vi "RenameTerminals.vi"(6 "Dynamic Dispatch":bool, 8 "error in (no error)":errorcluster, 11 "CreateInterface in":refnum<class "CreateInterface.lvclass">) -> (0 "error out":errorcluster)   [LabVIEW 2020, in "Mermaid.lvlib" / "CreateInterface.lvclass"]
uses:
  CreateInterface.lvclass
  CreateInterface.lvclass/CreateInterface.ctl
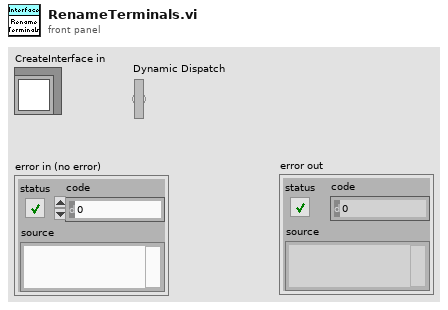
[diagram p1: front panel]
types:
  T1 = enum16{"Invalid Wire Rule", "Required", "Recommended", "Optional", "Dynamic Dispatch"}
  T2 = enum16{"Invalid Wire Rule", "Required", "Recommended", "Optional", "Dynamic Dispatch"}[]
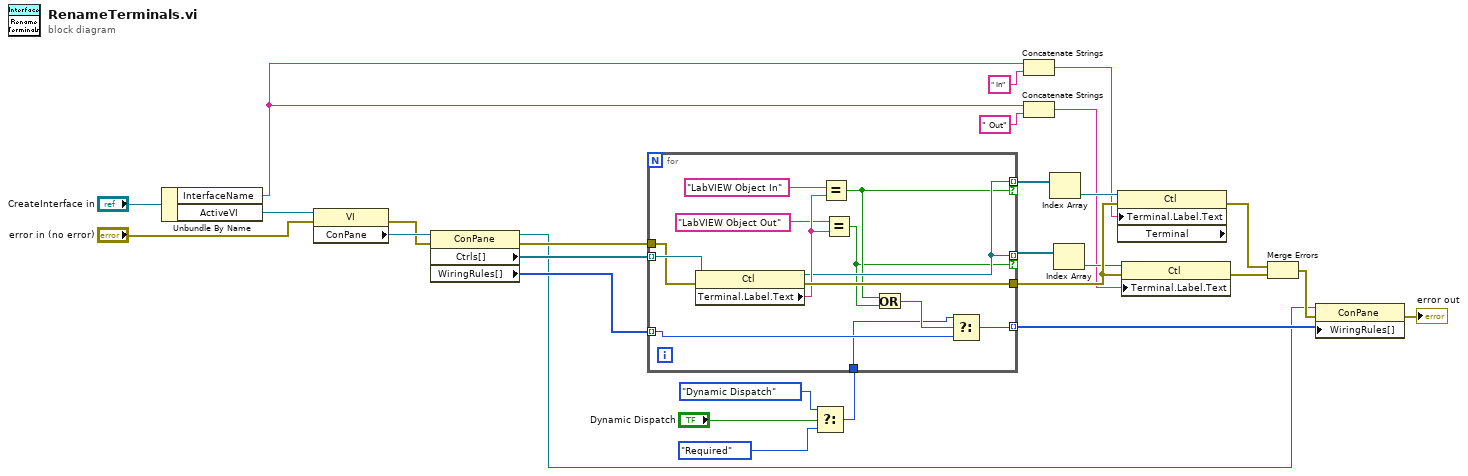
[diagram p0: block diagram]
diagram:
  n1 = Unbundle By Name("CreateInterface in") -> ("InterfaceName"=w6:string, "ActiveVI"=w26:refnum<vi>)
  n2 = property class="VI"(reference=w26, error in="error in (no error)") -> (error out=w11:errorcluster, "ConPane"=w21:refnum<vi>)  [unwired: 1 out]
  n3 = property class="ConPane"(reference=w21, error in=w11) -> (reference out=w1:refnum<vi>, error out=w13:errorcluster, "Ctrls[]"=w12:refnum<vi>[], "WiringRules[]"=w22:T2)
  n4 = Select(t=T1."Dynamic Dispatch" ("Wire Rule"), s="Dynamic Dispatch", f=T1."Required" ("Wire Rule")) -> (s? t:f=w2:T1)
  n5 = for {
    tunnel: w12 -> [w41] mode=indexing
    tunnel: w13 -> [w40]
    tunnel: [w39] -> w18
    tunnel: [w35] -> w14 mode=indexing if=w34
    tunnel: [w35] -> w17 mode=indexing if=w33
    tunnel: w22 -> [w31] mode=indexing
    tunnel: [w30] -> w24 mode=indexing
    tunnel: w2 -> [w29]
    n6 = property class="Ctl"(reference=w41, error in=w40) -> (reference out=w35:refnum<vi>, error out=w39:errorcluster, "Terminal.Label.Text"=w38:string)
    n7 = Equal?(x="LabVIEW Object In" ("name/order"), y=w38) -> (x = y?=w34:bool)
    n8 = Equal?(x="LabVIEW Object Out" ("name/order"), y=w38) -> (x = y?=w33:bool)
    n9 = Or(x=w34, y=w33) -> (x .or. y?=w32:bool)
    n10 = Select(t=w29, s=w32, f=w31) -> (s? t:f=w30:T1)
  }
  n11 = Concatenate Strings(w6, " In" ("string")) -> (w8:string)
  n12 = Concatenate Strings(w6, " Out" ("string")) -> (w7:string)
  n13 = Index Array(array=w14) -> (element=w15:refnum<vi>)  [unwired: 1 in]
  n14 = Index Array(array=w17) -> (element=w16:refnum<vi>)  [unwired: 1 in]
  n15 = property class="Ctl" props=["Terminal", "Label", "Text", "Terminal"](reference=w15, error in=w18, "Terminal.Label.Text"=w8) -> (error out=w20:errorcluster)  [unwired: 2 out]
  n16 = property class="Ctl"(reference=w16, error in=w18, "Terminal.Label.Text"=w7) -> (error out=w19:errorcluster)  [unwired: 1 out]
  n17 = Merge Errors(w20, w19) -> (w23:errorcluster)
  n18 = property class="ConPane"(reference=w1, error in=w23, "WiringRules[]"=w24) -> (error out=→"error out":errorcluster)  [unwired: 1 out]
